vi "Open.vi"(8 "error in (no error)":errorcluster caption="entrée d'erreur (pas d'erreur)", 11 "Class Printer_CAB en entrée":refnum<class "Class Printer_CAB.lvclass">) -> (0 "error out":errorcluster caption="sortie d'erreur", 3 "Class Printer_CAB en sortie":refnum<class "Class Printer_CAB.lvclass">)   [LabVIEW 2020, in "Library Instrument & Equipement.lvlib" / "Library Printer.lvlib" / "Class Printer_CAB.lvclass"]
uses:
  Class Printer_CAB.lvclass
  C:/Users/ngarcin/OneDrive - Altyor/Standard TB/Class/Printer/Printer (Default)/Class Printer (Default).lvclass
  <vilib>/Instr/_visa.llb/VISA Set IO Buffer Mask.ctl
  Class Printer_CAB.lvclass/Class Printer_CAB.ctl
  <vilib>/Instr/_visa.llb/VISA Configure Serial Port (Instr).vi
  Printer (Default)/Class Printer (Default).lvclass
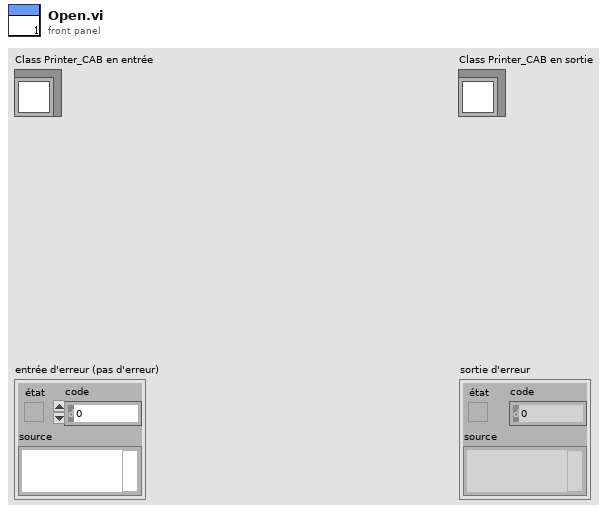
[diagram p1: front panel]
types:
  T1 = typedef "VISA Set IO Buffer Mask.ctl" = u16
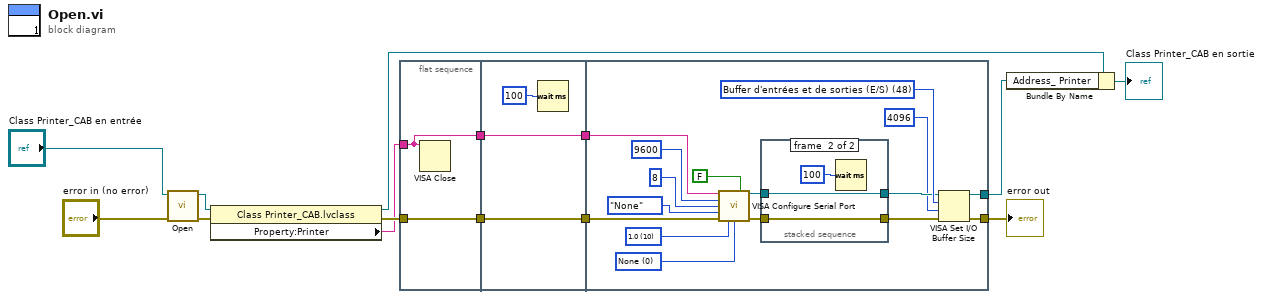
[diagram p0: block diagram]
diagram:
  n1 = call-parent "Open.vi"("error in (no error)"="error in (no error)", "Class Printer (Default) en entrée"="Class Printer_CAB en entrée") -> ("error out"=w6:errorcluster, "Class Printer (Default) en sortie"=w7:refnum<class "Class Printer_CAB.lvclass">)  [unwired: 8 in]
  n2 = property class="Class Printer_CAB.lvclass"(reference=w7, error in=w6) -> (reference out=w1:refnum<class "Class Printer_CAB.lvclass">, error out=w3:errorcluster, "Property:Printer"=w2:string)
  n3 = flat-sequence {
    tunnel: w2 -> [w16]
    tunnel: [w16] -> w9
    tunnel: [w15] -> w4
    tunnel: w3 -> [w15]
    tunnel: w9 -> [w19]
    tunnel: [w19] -> w8
    tunnel: [w17] -> w5
    tunnel: w4 -> [w17]
    tunnel: [w35] -> w12
    tunnel: [w33] -> w10
    tunnel: w8 -> [w34]
    tunnel: w5 -> [w20]
    frame #0 {
      n4 = VISA Close(VISA resource name=w16) -> ()  [unwired: 1 in, 1 out]
    }
    frame #1 {
      n5 = Wait (ms)(milliseconds to wait=u32 100 ("attente (ms)")) -> ()  [unwired: 1 out]
    }
    frame #2 {
      w31 = T1 48 items=["Buffer d'entrées (E/S)"=16, "Buffer de sorties (E/S)"=32, "Buffer d'entrées et de sorties (E/S)"=48] ("Mask")
      w21 = u16 0 items=["None", "XON/XOFF", "RTS/CTS", "XON/XOFF & RTS/CTS", "DTR/DSR", "XON/XOFF & DTR/DSR"] ("flow control (0:none)")
      w22 = u16 10 items=["1.0"=10, "1.5"=15, "2.0"=20] ("stop bits (10: 1 bit)")
      n6 = call-poly "VISA Configure Serial Port"("VISA resource name"=w34, "Enable Termination\nChar (T)"=FALSE ("Enable Termination\nChar (T)"), "baud rate (9600)"=9600, "data bits (8)"=u16 8, "parity (0:none)"=enum16{"None", "Odd", "Even", "Mark", "Space"}."None", "error in (no error)"=w20, "stop bits (10: 1 bit)"=w22, "flow control (0:none)"=w21) -> ("VISA resource name out"=w26:refnum<visa-resource-name>, "error out"=w29:errorcluster)  [unwired: 6 in]
      n7 = stacked-sequence {
        tunnel: w26 -> [_ w38]
        tunnel: [_ w38] -> w27
        tunnel: [_ w37] -> w28
        tunnel: w29 -> [_ w37]
        frame #0 {
        }
        frame #1 {
          n8 = Wait (ms)(milliseconds to wait=u32 100) -> ()  [unwired: 1 out]
        }
      }
      n9 = VISA Set I/O Buffer Size(VISA resource name=w27, mask (16)=w31, size (4096)=u32 4096 ("taille (4096)"), error in (no error)=w28) -> (VISA resource name out=w33:refnum<visa-resource-name>, error out=w35:errorcluster)
    }
  }
  n10 = Bundle By Name(cluster=w1, "Address_ Printer"=w10) -> (→"Class Printer_CAB en sortie":refnum<class "Class Printer_CAB.lvclass">)
  "error out" <- w12
